vi "VI_find_salt.vi"(7 "Verify salt (T)":bool=TRUE, 8 "error in (no error)":errorcluster, 9 "CONP block":string, 10 "VCTP block":string, 11 "Hashes":T1) -> (0 "error out":errorcluster, 3 "Salt":string)   [LabVIEW 2020]
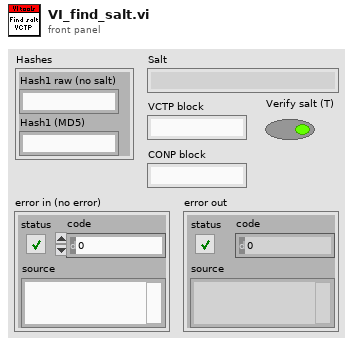
[diagram p1: front panel]
types:
  T1 = cluster{"Hash1 raw (no salt)":string, "Hash1 (MD5)":string}
  T2 = enum16{"big-endian, network order", "native, host order", "little-endian"}
  T3 = cluster{"Numbers":i32, "Strings":i32, "Paths":i32}
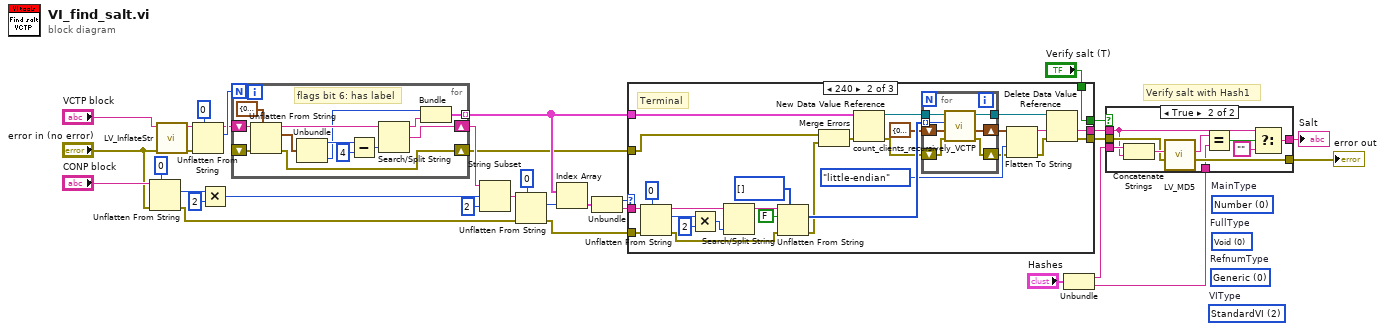
[diagram p0: block diagram]
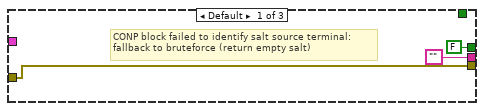
[diagram p3: hidden frame]
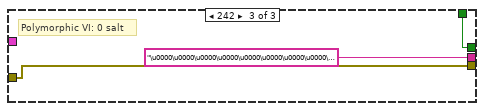
[diagram p4: hidden frame]
diagram:
  (unwired) u16 2 items=["DialogVI", "ProbeVI", "StandardVI", "ClipboardVI", "GlobalVI", "HierarchyVI", "ControlVI", "ConfigVI", "PxCallerVI", "PxCalleeVI", "SubSystemVI", "PolyVI", "FacadeVI", "MethodVI", "StatechartVI"]  # VIType
  (unwired) u8 0 items=["Generic"=0, "DataLog"=1, "ByteStream"=2, "Device"=3, "Occurrence"=4, "TCPNetConn"=5, "AutoRef"=7, "LVObjCtl"=8, "Menu"=9, "Imaq"=11, "DataSocket"=13, "VisaRef"=14, "IVIRef"=15, "UDPNetConn"=16, "NotifierRef"=17, "Queue"=18, "IrdaNetConn"=19, "UsrDefined"=20, "UsrDefndTag"=21, "EventReg"=23, "DotNet"=24, "UserEvent"=25, "Callback"=27, "UsrDefTagFlt"=29, "UDClassInst"=30, "BluetoothCon"=31, "DataValueRef"=32, "FIFORef"=33, "TDMSFile"=34]  # RefnumType
  (unwired) u8 0 items=["Void"=0, "NumberI8"=1, "NumberI16"=2, "NumberI32"=3, "NumberI64"=4, "NumberU8"=5, "NumberU16"=6, "NumberU32"=7, "NumberU64"=8, "NumberSGL"=9, "NumberDBL"=10, "NumberEXT"=11, "NumberCSG"=12, "NumberCDB"=13, "NumberCXT"=14, "UnitI8"=17, "UnitI16"=18, "UnitI32"=19, "UnitI64"=20, "UnitU8"=21, "UnitU16"=22, "UnitU32"=23, "UnitU64"=24, "UnitSGL"=25, "UnitDBL"=26, "UnitEXT"=27, "UnitCSG"=28, "UnitCDB"=29, "UnitCXT"=30, "BoolU16"=32, "Bool"=33, "String"=48, "String2"=49, "Path"=50, "Picture"=51, "CString"=52, "PascalString"=53, "Tag"=55, "SubString"=63, "Array"=64, "ArrayDataPtr"=65, "SubArray"=79, "Cluster"=80, "LVVariant"=83, "MeasureData"=84, "ComplexFixedPt"=94, "FixedPoint"=95, "Block"=96, "TypeBlock"=97, "VoidBlock"=98, "AlignedBlock"=99, "RepeatedBlock"=100, "AlignmntMarker"=101, "Refnum"=112, "Set"=115, "Map"=116, "PointerNumber"=128, "PointerNumberI8"=129, "PointerNumberI16"=130, "PointerNumberI32"=131, "PointerNumberI64"=132, "PointerNumberU8"=133, "PointerNumberU16"=134, "PointerNumberU32"=135, "PointerNumberU64"=136, "PointerNumberSGL"=137, "PointerNumberDBL"=138, "PointerNumberEXT"=139, "PointerNumberCSG"=140, "PointerNumberCDB"=141, "PointerNumberCXT"=142, "ArrayInterfc"=160, "InterfcToData"=161, "Terminal"=240, "TypeDef"=241, "PolyVI"=242]  # FullType
  (unwired) u8 0 items=["Number"=0, "Unit"=1, "Bool"=2, "Blob"=3, "Array"=4, "Cluster"=5, "Block"=6, "Refnum"=7, "NumberPointer"=8, "Terminal"=15]  # MainType
  # "Verify salt with Hash1"
  n1 = Unflatten From String(type=i16 0, binary string="CONP block", error in (no error)="error in (no error)") -> (value=w24:i16, error out=w17:errorcluster)  [unwired: 2 in, 1 out]
  n2 = call "LV_InflateStr.vi"("error in (no error)"="error in (no error)", "Deflated string with size header"="VCTP block") -> ("error out"=w28:errorcluster, "Inflated string"=w30:string)  [unwired: 8 in]
  n3 = Unflatten From String(type=0, binary string=w30, error in (no error)=w28) -> (rest of the binary string=w31:string, value=w32:i32)  [unwired: 2 in, 1 out]
  n4 = Multiply(x=w24, y=i16 2) -> (x*y=w21:i16)
  n5 = for {
    N: w32 -> [_]
    shift-right: [w41] -> w22
    shift-left: w31 -> [w46]
    tunnel: [w39] -> w11 mode=indexing
    shift-right: [w34] -> w10
    shift-left: _ -> [w36]
    # "flags bit 6: has label"
    n6 = Unflatten From String(type=cluster{"length":i16, "flags":u8, "type":u8} {"length"=0, "flags"=0, "type"=0}, binary string=w46, error in (no error)=w36) -> (rest of the binary string=w43:string, value=w44:cluster{"length":i16, "flags":u8, "type":u8}, error out=w34:errorcluster)  [unwired: 2 in]
    n7 = Unbundle(w44) -> ("length"=w40:i16, "type"=w35:u8)  [unwired: 1 out]
    n8 = Subtract(x=w40, y=i16 4) -> (x-y=w42:i16)
    n9 = Search/Split String(string=w43, offset (0)=w42) -> (substring before match=w37:string, match + rest of string=w41:string)  [unwired: 1 in, 1 out]
    n10 = Bundle("type"=w35, w37) -> (w39:cluster{"type":u8, string})  [unwired: 1 in]
  }
  n11 = String Subset(string=w22, offset (0)=w21, length (rest)=2 ("length (rest)")) -> (substring=w18:string)
  n12 = Unflatten From String(type=i16 0, binary string=w18, error in (no error)=w17) -> (value=w16:i16, error out=w12:errorcluster)  [unwired: 2 in, 1 out]
  n13 = Index Array(array=w11, index=w16) -> (element=w15:cluster{"type":u8, string})
  n14 = Unbundle(w15) -> ("type"=w14:u8, w13:string)
  n15 = case shown="240" w14 {
    tunnel: w13 -> [_ w69 _]
    tunnel: w12 -> [_ w68 _]
    tunnel: w11 -> [_ w65 _]
    tunnel: w10 -> [w49 w64 w85]
    tunnel: ["" w52 "\u0000\u0000\u0000\u0000\u0000\u0000\u0000\u0000\u0000\u0000\u0000\u0000" ("Salt")] -> w8
    tunnel: [w49 w51 w85] -> w7
    tunnel: [FALSE ("Verify salt (T)") w50 w84] -> w4
    tunnel: "Verify salt (T)" -> [_ w50 w84]
    frame Default {
      # "CONP block failed to identify salt source terminal:\nfallback to bruteforce (return empty salt)"
    }
    frame 240 {
      # "Terminal"
      n16 = Unflatten From String(type=i16 0, binary string=w69, error in (no error)=w68) -> (rest of the binary string=w73:string, value=w75:i16, error out=w67:errorcluster)  [unwired: 2 in]
      n17 = Multiply(x=w75, y=i16 2) -> (x*y=w72:i16)
      n18 = Search/Split String(string=w73, offset (0)=w72) -> (substring before match=w70:string)  [unwired: 1 in, 2 out]
      n19 = Unflatten From String(type=i16[] [] ("index"), binary string=w70, data includes array or string size? (T)=FALSE, error in (no error)=w67) -> (value=w63:i16[], error out=w62:errorcluster)  [unwired: 1 in, 1 out]
      n20 = Merge Errors(w64, w62) -> (w54:errorcluster)
      n21 = New Data Value Reference(data value=w65, error in=w54) -> (data value reference=w61:refnum<data-value>, error out=w60:errorcluster)
      n22 = for {
        tunnel: w63 -> [w82] mode=indexing
        shift-right: [w83] -> w56
        shift-left: T3 {"Numbers"=0, "Strings"=0, "Paths"=0} ("Control counts out") -> [w81]
        tunnel: [w80] -> w59
        shift-right: [w79] -> w55
        shift-left: w60 -> [w78]
        tunnel: w61 -> [w77]
        n23 = call "count_clients_recursively_VCTP.vi"("error in (no error)"=w78, "Control counts in (0)"=w81, "Type descriptor index"=w82, "VCTP type descriptor list"=w77) -> ("error out"=w79:errorcluster, "Control counts out"=w83:T3, "Type descriptor list dup"=w80:refnum<data-value>)  [unwired: 5 in]
      }
      n24 = Flatten To String(anything=w56, byte order (0:big-endian, network order)=T2."little-endian", error in (no error)=w55) -> (data string=w52:string, error out=w53:errorcluster)  [unwired: 1 in, 1 out]
      n25 = Delete Data Value Reference(data value reference=w59, error in=w53) -> (error out=w51:errorcluster)  [unwired: 1 out]
    }
    frame 242 {
      # "Polymorphic VI: 0 salt"
    }
  }
  n26 = Unbundle("Hashes") -> ("Hash1 raw (no salt)"=w6:string, "Hash1 (MD5)"=w5:string)
  n27 = case shown="True" w4 {
    tunnel: [w88 w98] -> w1
    tunnel: w8 -> [w87 w90]
    tunnel: w5 -> [_ w97]
    tunnel: w6 -> [_ w96]
    tunnel: w7 -> [w88 w94]
    tunnel: [w87 w89] -> w2
    frame False {
    }
    frame True {
      n28 = Concatenate Strings(w96, w90) -> (w95:string)
      n29 = call "LV_MD5.vi"("error in (no error)"=w94, "Input string"=w95) -> ("error out"=w98:errorcluster, "MD5 digest (16-bytes)"=w93:string)  [unwired: 8 in]
      n30 = Equal?(x=w93, y=w97) -> (x = y?=w91:bool)
      n31 = Select(t=w90, s=w91, f="") -> (s? t:f=w89:string)
    }
  }
  "Salt" <- w2
  "error out" <- w1
